vi "isLastDataReceived.vi"(8 "error in (no error)":errorcluster, 10 "Board":u16, 11 "identifier":string) -> (0 "error out":errorcluster, 1 "LastDataReceived out":u8, 3 "function return":bool)   [LabVIEW 2015, in "XGL_DPP.lvlib"]
uses:
  XGL_DPP.lvlib
  DANTE/DANTE-v2.0.8.9/DANTE v2.0.8.9/Examples/Labview2013/libs/XGL_DPP.dll
panel:
  in  "LastDataReceived in":u8
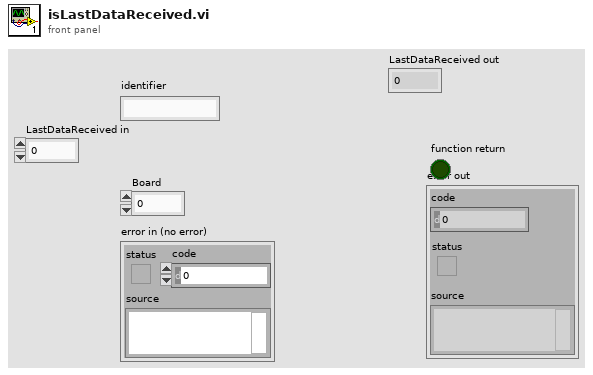
[diagram p1: front panel]
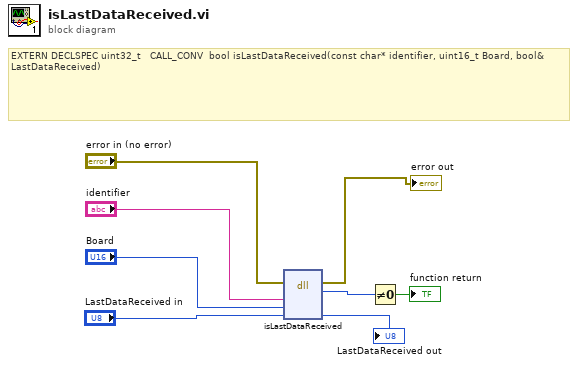
[diagram p0: block diagram]
diagram:
  # "EXTERN DECLSPEC uint32_t   CALL_CONV  bool isLastDataReceived(const char* identifier, uint16_t Board, bool& LastDataReceived)"
  n1 = dll-call lib="D:/DANTE/DANTE-v2.0.8.9/DANTE v2.0.8.9/Examples/Labview2013/libs/XGL_DPP.dll" fn="isLastDataReceived"(error in="error in (no error)", "Identifier"="identifier", "Board"="Board", "LastDataReceived"="LastDataReceived in") -> (error out=→"error out":errorcluster, "return type"=w3:u32, "LastDataReceived"=→"LastDataReceived out":u8)  [unwired: 4 in, 1 out]
  n2 = Not Equal To 0?(x=w3) -> (x != 0?=→"function return":bool)
